vi "Init Device.vi"(8 "error in (no error)":errorcluster, 11 "Stage Controller in":refnum<class "Stage Controller.lvclass">) -> (0 "error out":errorcluster, 3 "Stage Controller out":refnum<class "Stage Controller.lvclass">)   [LabVIEW 2018, in "Stage Controller.lvlib" / "Stage Controller.lvclass"]
uses:
  Stage Controller.lvclass
  Stage Controller.lvclass/Stage Controller.ctl
  <instrlib>/ASI TG-1000/Public/Utility/Baud Rate.ctl
  <vilib>/Instr/_visa.llb/VISA Configure Serial Port (Instr).vi
  Device/Device.lvclass
  <instrlib>/ASI TG-1000/ASI TG-1000.lvlib
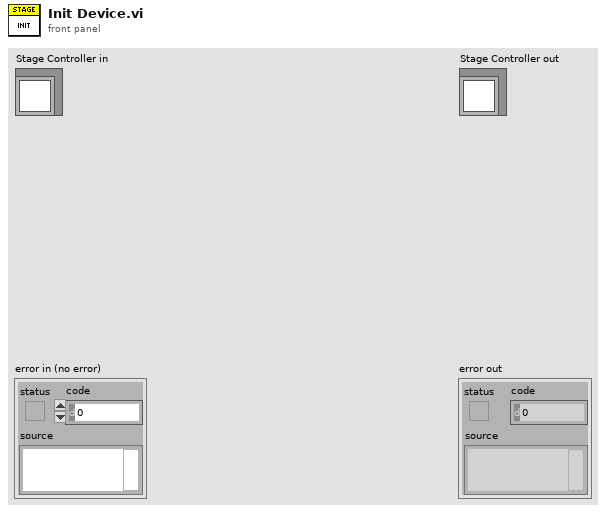
[diagram p1: front panel]
types:
  T1 = enum16{"Disabled", "ESP301", "Ti2", "Ludl", "ASI"}
  T2 = typedef "Stage Controller.lvlib/ASI TG-1000.lvlib/Baud Rate.ctl" = u32
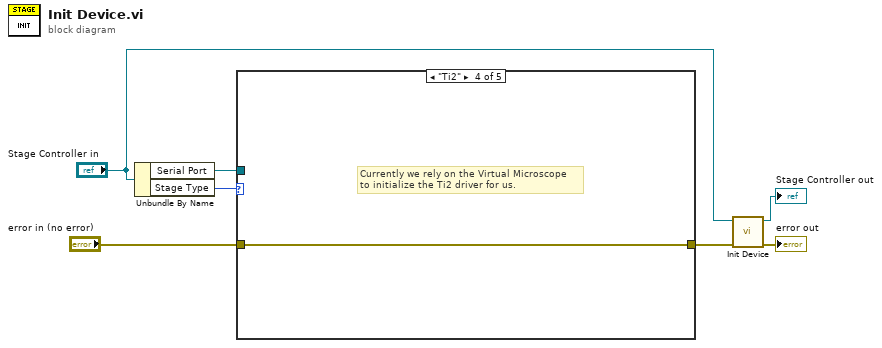
[diagram p0: block diagram]
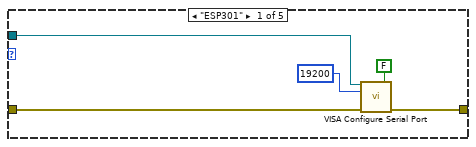
[diagram p2: hidden frame]
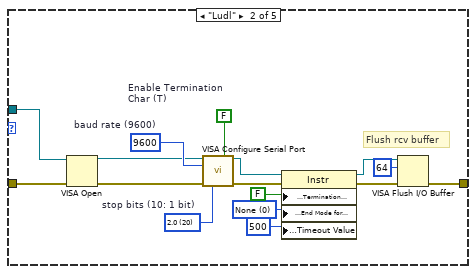
[diagram p3: hidden frame]
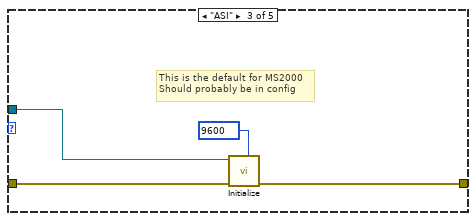
[diagram p4: hidden frame]
diagram:
  n1 = Unbundle By Name("Stage Controller in") -> ("Serial Port"=w2:refnum<visa-resource-name>, "Stage Type"=w1:T1)
  n2 = case shown="\"Ti2\"" w1 {
    tunnel: "error in (no error)" -> [w12 w25 w32 w33 w34]
    tunnel: [w11 w20 w29 w33 w34] -> w4
    tunnel: w2 -> [w8 w22 w31 _ _]
    frame "ESP301" {
      n3 = call-poly "VISA Configure Serial Port"("VISA resource name"=w8, "Enable Termination\nChar (T)"=FALSE ("Enable Termination\nChar (T)"), "baud rate (9600)"=u32 19200, "error in (no error)"=w12) -> ("error out"=w11:errorcluster)  [unwired: 10 in, 1 out]
    }
    frame "Ludl" {
      w18 = u16 0 items=["None", "LastBit", "TermChar"] ("Serial Settings:Serial End Mode for Reads")
      w26 = u16 20 items=["1.0"=10, "1.5"=15, "2.0"=20]  # stop bits (10: 1 bit)
      w28 = FALSE  # Enable Termination Char (T)
      w27 = u32 9600  # baud rate (9600)
      # "Flush rcv buffer"
      n4 = VISA Open(error in (no error)=w25, VISA resource name=w22) -> (VISA resource name=w23:refnum<visa-resource-name>, error out=w24:errorcluster)  [unwired: 3 in]
      n5 = call-poly "VISA Configure Serial Port"("VISA resource name"=w23, "Enable Termination\nChar (T)"=w28, "baud rate (9600)"=w27, "error in (no error)"=w24, "stop bits (10: 1 bit)"=w26) -> ("VISA resource name out"=w16:refnum<visa-resource-name>, "error out"=w13:errorcluster)  [unwired: 9 in]
      n6 = property class="Instr"(reference=w16, error in=w13, "Message Based Settings:Termination Character Enable"=FALSE, "Serial Settings:End Mode for Reads"=w18, "General Settings:Timeout Value"=u32 500) -> (reference out=w15:refnum<visa-resource-name>, error out=w14:errorcluster)
      n7 = VISA Flush I/O Buffer(VISA resource name=w15, mask (16)=u16 64, error in (no error)=w14) -> (error out=w20:errorcluster)  [unwired: 1 out]
    }
    frame "ASI" {
      w30 = T2 9600 items=["9600"=9600, "19200"=19200, "28800"=28800, "115200"=115200] ("Baud Rate (115200)")
      # "This is the default for MS2000\nShould probably be in config"
      n8 = call <instrlib>:"Initialize.vi"("Baud Rate (115200)"=w30, "error in (no error)"=w32, "VISA resource name"=w31) -> ("error out"=w29:errorcluster)  [unwired: 7 in, 1 out]
    }
    frame "Ti2" {
      # "Currently we rely on the Virtual Microscope\nto initialize the Ti2 driver for us."
    }
    frame "Disabled", Default {
    }
  }
  n9 = call-parent "Init Device.vi"("error in (no error)"=w4, "Device in"="Stage Controller in") -> ("error out"=→"error out":errorcluster, "Device out"=→"Stage Controller out":refnum<class "Stage Controller.lvclass">)  [unwired: 8 in]
